vi "sim_pmt.vi"(4 "A":dbl=1.0, 6 "eff":dbl=0.25, 7 "N":i32=600, 8 "tau":dbl=142.0, 9 "sigma":dbl=10.0, 10 "dx":dbl=1.0 format="%#_13g", 11 "x0":dbl=-100.0) -> (2 "y":dbl[](array[numeric])=[1.9287498479639178e-22, 5.216736662027038e-22, 1.3969439431470991e-21, 3.703531977652345e-21, 9.72098502030078e-21, 2.5261637809256925e-20, 6.499347972070893e-20, 1.6555226620987744e-19, 4.175010055850514e-19, 1.04240617839016e-18, 2.576757109154981e-18, 6.306189893986447e-18, 1.5279799682873048e-17, 3.665433395601045e-17, 8.705426622296251e-17, 2.0469717131642043e-16, 4.765304735299088e-16, 1.0983141298285972e-15, 2.5062218871452745e-15, 5.6619955169489504e-15, 1.2664165549094176e-14, 2.804404738222797e-14, 6.148396412704756e-14, 1.3345660848219891e-13, 2.867975008888098e-13, 6.101936677605324e-13, 1.2853372251336503e-12, 2.680547637312607e-12, 5.5346100717010135e-12, 1.1313776200065328e-11, 2.289734845645553e-11, 4.5879624871392916e-11, 9.101470764487935e-11, 1.7875588711279812e-10, 3.475891281239922e-10, 6.691586091292782e-10, 1.2754076295260442e-09, 2.406722436301052e-09, 4.49634946228087e-09, 8.316702456828333e-09, 1.522997974471263e-08, 2.761242456828035e-08, 4.956405319172498e-08, 8.808179196460557e-08, 1.5497531357028967e-07, 2.699578503363014e-07, 4.6557157157830866e-07, 7.949393615349141e-07, 1.3438122776315214e-06, 2.2490559670323425e-06, 3.726653172078671e-06, 6.113567966371402e-06, 9.929504305851081e-06, 1.5966783897804747e-05, 2.5419346516199247e-05, 4.006529739295107e-05, 6.252150377482026e-05, 9.659341372218401e-05, 0.00014774836023203364, 0.00022374579372062055, 0.00033546262790251185, 0.0004979554215032735, 0.0007318024188804728, 0.0010647662366679205, 0.001533810679324463, 0.002187491118182885, 0.0030887154082367687, 0.004317840007633078, 0.005976022895005943, 0.008188701014374083, 0.011108996538242306, 0.014920786069067842, 0.019841094744370288, 0.026121409853918233, 0.034047454734599344, 0.04393693362340742, 0.056134762834133725, 0.07100535373963698, 0.08892161745938634, 0.11025052530448522, 0.1353352832366127, 0.1644744565771549, 0.19789869908361465, 0.23574607655586352, 0.27803730045319414, 0.32465246735834974, 0.37531109885139957, 0.42955735821073915, 0.4867522559599717, 0.5460744266397094, 0.6065306597126334, 0.6669768108584744, 0.7261490370736909, 0.7827045382418681, 0.835270211411272, 0.8824969025845955, 0.9231163463866358, 0.9559974818331, 0.9801986733067553, 0.9950124791926823, 1.25, 1.2432581004527816, 1.2267022272060057, 1.2007711933552672, 1.1661723547264784, 1.123847261749892, 1.0749268908206204, 1.0206794233182925, 0.9624539298340817, 0.9016234304988917, 0.8395306431895039, 0.7774393292469436, 0.7164935519020325, 0.657686441171688, 0.6018392825599493, 0.549590986148953, 0.5013973098231934, 0.4575386537187317, 0.4181348435183134, 0.3831650905736379, 0.35249125243750024, 0.32588259924293844, 0.3030404900932062, 0.2836216439816156, 0.267259015078684, 0.2535796182694965, 0.24221896870501314, 0.23283207711088139, 0.22510116680154815, 0.21874044249997526, 0.21349834548108462, 0.20915777967334567, 0.20553479803807054, 0.20247620846081113, 0.1998565045464241, 0.19757445935252493, 0.1955496479411705, 0.19371909445812904, 0.19203417601001516, 0.19045786174415458, 0.1889623224662098, 0.18752691382132963, 0.18613651360422623, 0.18478017971529853, 0.18345008797568668, 0.18214070677818295, 0.18084816685156144, 0.17956978795328984, 0.17830372904758776, 0.1770487337057488, 0.1758039475556503, 0.17456878927836056, 0.17334286072721433, 0.17212588516622737, 0.17091766540284734, 0.16971805578245663, 0.168526943698985, 0.16734423754450112, 0.16616985895450573, 0.1650037378796452, 0.16384580949201014, 0.162696012266431, 0.1615542868044931, 0.1604205751219807, 0.1592948202218085, 0.15817696584061583, 0.157066956299691, 0.1559647364178046, 0.15487025146033528, 0.15378344710941852, 0.1527042694461285, 0.15163266493947214, 0.1505685804391951, 0.14951196317070164, 0.1484627607311352, 0.14742092108609436, 0.14638639256669508, 0.14535912386682462, 0.14433906404050334, 0.14332616249931096, 0.14232036900985437, 0.14132163369126458, 0.14032990701271744, 0.1393451397909746, 0.1383672831879428, 0.1373962887082515, 0.13643210819684728, 0.13547469383660565, 0.1345239981459596, 0.13357997397654467, 0.13264257451086087, 0.13171175325995063, 0.13078746406109337, 0.1298696610755161, 0.12895829878612006, 0.12805333199522348, 0.12715471582231996, 0.12626240570185276, 0.12537635738100453, 0.12449652691750278, 0.12362287067744056, 0.12275534533311253, 0.12189390786086615, 0.12103851553896804, 0.12018912594548517, 0.1193456969561811, 0.11850818674242683, 0.1176765537691264, 0.11685075679265702, 0.1160307548588236, 0.11521650730082776, 0.11440797373725096, 0.11360511407005193, 0.1128078884825779, 0.11201625743759017, 0.11123018167530312, 0.11044962221143731, 0.10967454033528602, 0.10890489760779555, 0.1081406558596588, 0.10738177718942235, 0.1066282239616068, 0.10587995880484032, 0.10513694461000518, 0.10439914452839749, 0.10366652196989969, 0.10293904060116589, 0.10221666434382001, 0.10149935737266652, 0.10078708411391372, 0.10007980924340955, 0.0993774976848897, 0.09868011460823806, 0.09798762542775939, 0.0972999958004641, 0.09661719162436501, 0.09593917903678618, 0.09526592441268349, 0.09459739436297705, 0.09393355573289539, 0.09327437560033107, 0.0926198212742081, 0.09196986029286058, 0.09132446042242282, 0.09068358965523078, 0.09004721620823468, 0.08941530852142278, 0.08878783525625616, 0.0881647652941146, 0.08754606773475325, 0.0869317118947702, 0.08632166730608473, 0.08571590371442639, 0.0851143910778345, 0.08451709956516827, 0.08392399955462743, 0.0833350616322831, 0.0827502565906191, 0.08216955542708343, 0.08159292934264993, 0.08102034974039005, 0.08045178822405458, 0.07988721659666545, 0.0793266068591173, 0.07876993120878888, 0.0782171620381643, 0.07766827193346378, 0.07712323367328416, 0.07658202022724891, 0.07604460475466757, 0.07551096060320459, 0.07498106130755759, 0.07445488058814488, 0.0739323923498021, 0.07341357068048812, 0.07289838984999991, 0.07238682430869656, 0.07187884868623211, 0.07137443779029741, 0.07087356660537074, 0.07037621029147711, 0.0698823441829565, 0.06939194378724046, 0.06890498478363756, 0.06842144302212716, 0.06794129452216174, 0.06746451547147767, 0.06699108222491419, 0.06652097130324086, 0.06605415939199304, 0.0655906233403157, 0.06513034015981535, 0.0646732870234198, 0.06421944126424624, 0.06376878037447704, 0.0633212820042435, 0.06287692396051747, 0.06243568420601071, 0.06199754085808197, 0.06156247218765177, 0.06113045661812477, 0.06070147272431971, 0.06027549923140684, 0.05985251501385289, 0.05943249909437331, 0.05901543064289194, 0.05860128897550802, 0.05819005355347037, 0.05778170398215878, 0.05737622001007262, 0.05697358152782646, 0.056573768567152766, 0.05617676129991164, 0.055782540037107455, 0.0553910852279124, 0.05500237745869686, 0.05461639745206672, 0.05423312606590721, 0.05385254429243366, 0.05347463325724882, 0.053099374218406784, 0.052726748565483546, 0.052356737818654034, 0.051989323627775606, 0.05162448777147804, 0.05126221215625983, 0.05090247881559093, 0.05054526990902163, 0.050190567721297895, 0.04983835466148272, 0.04948861326208375, 0.04914132617818706, 0.048796476186596896, 0.04845404618498154, 0.04811401919102513, 0.04777637834158547, 0.04744110689185774, 0.04710818821454399, 0.04677760579902863, 0.04644934325055953, 0.04612338428943498, 0.04579971275019635, 0.04547831258082632, 0.04515916784195286, 0.044842262706058726, 0.044527581456696504, 0.04421510848770919, 0.04390482830245621, 0.043596725513044915, 0.0432907848395674, 0.04298699110934278, 0.04268532925616464, 0.042385784319553914, 0.04208834144401693, 0.04179298587830866, 0.041499702974701146, 0.04120847818825709, 0.040919297076108516, 0.04063214529674048, 0.04034700860927983, 0.04006387287278897, 0.03978272404556454, 0.039503548184441024, 0.03922633144409931, 0.03895106007637999, 0.03867772042960159, 0.03840629894788351, 0.03813678217047375, 0.03786915673108132, 0.0376034093572134, 0.037339526869517074, 0.037077496181125734, 0.03681730429701006, 0.03655893831333352, 0.036302385416812494, 0.03604763288408073, 0.03579466808105841, 0.035543478462325556, 0.035294051570499856, 0.03504637503561887, 0.03480043657452655, 0.03455622399026408, 0.03431372517146501, 0.034072928091754544, 0.033833820809153176, 0.0335963914654844, 0.03336062828578669, 0.03312651957772941, 0.032894053731033115, 0.032663219216893594, 0.032434004587410255, 0.03220639847501826, 0.03198038959192488, 0.031755966729549605, 0.03153311875796834, 0.03131183462536134, 0.031092103357465258, 0.030873914057028714, 0.030657255903272018, 0.03044211815135042, 0.030228490131821318, 0.030016361250115038, 0.029805720986009508, 0.029596558893108423, 0.029388864598323267, 0.029182627801358774, 0.028977838274202215, 0.028774485860616032, 0.028572560475634265, 0.02837205210506234, 0.028172950804980418, 0.02797524670125031, 0.027778929989025692, 0.02758399093226594, 0.0273904198632532, 0.027198207182113018, 0.027007343356338146, 0.02681781892031591, 0.02662962447485866, 0.02644275068673773, 0.026257188288220486, 0.02607292807661079, 0.025889960913792507, 0.025708277725776434, 0.02552786950225016, 0.02534872729613133, 0.02517084222312382, 0.024994205461277244, 0.02481880825054933, 0.024644641892371585, 0.024471697749217796, 0.02429996724417578, 0.024129441860521905, 0.02396011314129881, 0.02379197268889597, 0.023625012164633166, 0.023459223288347052, 0.0232945978379804, 0.023131127649174438, 0.02296880461486386, 0.02280762068487486, 0.02264756786552579, 0.02248863821923084, 0.02233082386410628, 0.022174116973579655, 0.022018509776001564, 0.02186399455426031, 0.0217105636453991, 0.0215582094402361, 0.021406924382986983, 0.02125670097089028, 0.021107531753835243, 0.020959409333992412, 0.02081232636544667, 0.02066627555383301, 0.0205212496559747, 0.02037724147952414, 0.02023424388260614, 0.02009224977346369, 0.019951252110106326, 0.019811243899960838, 0.01967221819952452, 0.019534168114020773, 0.019397086797057234, 0.01926096745028616, 0.01912580332306735, 0.018991587712133294, 0.018858313961256788, 0.018725975460920773, 0.018594565647990603, 0.0184640780053885, 0.018334506061770412, 0.018205843391205, 0.01807808361285503, 0.017951220390660858, 0.017825247433026267, 0.017700158492506373, 0.017575947365497866, 0.017452607891931284, 0.017330133954965566, 0.01720851948068467, 0.01708775843779634, 0.016967844837333025, 0.01684877273235481, 0.016730536217654562, 0.01661312942946498, 0.016496546545167894, 0.016380781783005383, 0.016265829401793153, 0.016151683700635713, 0.016038339018643728, 0.015925789734653202, 0.015814030266946784, 0.015703055072976865, 0.01559285864909078, 0.015483435530257805, 0.015374780289798173, 0.0152668875391139, 0.015159751927421592, 0.015053368141487035, 0.014947730905361738, 0.014842834980121237, 0.014738675163605318, 0.014635246290159984, 0.014532543230381306, 0.01443056089086103, 0.014329294213933945, 0.01422873817742711, 0.014128887794410737, 0.014029738112950907, 0.013931284215863957, 0.013833521220472652, 0.013736444278363994, 0.013640048575148823, 0.013544329330222999, 0.01344928179653037, 0.013354901260327297, 0.01326118304094893, 0.013168122490577033, 0.013075714994009524, 0.012983955968431552, 0.012892840863188258, 0.012802365159559048, 0.012712524370533544, 0.012623314040589001, 0.012534729745469403, 0.012446767091965986, 0.012359421717699416, 0.012272689290903417, 0.01218656551020994, 0.01210104610443586, 0.01201612683237113, 0.011931803482568481, 0.011848071873134509, 0.011764927851522337, 0.011682367294325624, 0.011600386107074118, 0.01151898022403055, 0.011438145607989045, 0.01135787825007486, 0.011278174169545612, 0.011199029413593813, 0.011120440057150885, 0.011042402202692456, 0.010964911980045108, 0.010887965546194409, 0.010811559085094348, 0.010735688807478062, 0.010660350950669943, 0.010585541778398995, 0.010511257580613572, 0.010437494673297378, 0.010364249398286732, 0.0102915181230892, 0.010219297240703392, 0.010147583169440127, 0.010076372352744762, 0.010005661259020845, 0.009935446381454943, 0.00986572423784275, 0.009796491370416367, 0.00972774434567285, 0.009659479754203892, 0.009591694210526785, 0.009524384352916472, 0.009457546843238874, 0.009391178366785295, 0.009325275632108079, 0.009259835370857335, 0.009194854337618885, 0.00913032930975327, 0.009066257087235975, 0.009002634492498687, 0.00893945837027174, 0.008876725587427605, 0.00881443303282554, 0.008752577617157267, 0.008691156272793776, 0.008630165953633199, 0.008569603634949718, 0.008509466313243591, 0.008449751006092163, 0.00839045475200199, 0.008331574610261941, 0.00827310766079738, 0.008215051004025326, 0.008157401760710677, 0.008100157071823395, 0.008043314098396741, 0.007986870021386453, 0.007930822041530968, 0.007875167379212573, 0.007819903274319572, 0.007765026986109383, 0.00771053579307264, 0.007656426992798195, 0.007602697901839126, 0.007549345855579625, 0.007496368208102875, 0.007443762332059822], 3 "x":dbl[](array[numeric])=[-100.0, -99.0, -98.0, -97.0, -96.0, -95.0, -94.0, -93.0, -92.0, -91.0, -90.0, -89.0, -88.0, -87.0, -86.0, -85.0, -84.0, -83.0, -82.0, -81.0, -80.0, -79.0, -78.0, -77.0, -76.0, -75.0, -74.0, -73.0, -72.0, -71.0, -70.0, -69.0, -68.0, -67.0, -66.0, -65.0, -64.0, -63.0, -62.0, -61.0, -60.0, -59.0, -58.0, -57.0, -56.0, -55.0, -54.0, -53.0, -52.0, -51.0, -50.0, -49.0, -48.0, -47.0, -46.0, -45.0, -44.0, -43.0, -42.0, -41.0, -40.0, -39.0, -38.0, -37.0, -36.0, -35.0, -34.0, -33.0, -32.0, -31.0, -30.0, -29.0, -28.0, -27.0, -26.0, -25.0, -24.0, -23.0, -22.0, -21.0, -20.0, -19.0, -18.0, -17.0, -16.0, -15.0, -14.0, -13.0, -12.0, -11.0, -10.0, -9.0, -8.0, -7.0, -6.0, -5.0, -4.0, -3.0, -2.0, -1.0, 0.0, 1.0, 2.0, 3.0, 4.0, 5.0, 6.0, 7.0, 8.0, 9.0, 10.0, 11.0, 12.0, 13.0, 14.0, 15.0, 16.0, 17.0, 18.0, 19.0, 20.0, 21.0, 22.0, 23.0, 24.0, 25.0, 26.0, 27.0, 28.0, 29.0, 30.0, 31.0, 32.0, 33.0, 34.0, 35.0, 36.0, 37.0, 38.0, 39.0, 40.0, 41.0, 42.0, 43.0, 44.0, 45.0, 46.0, 47.0, 48.0, 49.0, 50.0, 51.0, 52.0, 53.0, 54.0, 55.0, 56.0, 57.0, 58.0, 59.0, 60.0, 61.0, 62.0, 63.0, 64.0, 65.0, 66.0, 67.0, 68.0, 69.0, 70.0, 71.0, 72.0, 73.0, 74.0, 75.0, 76.0, 77.0, 78.0, 79.0, 80.0, 81.0, 82.0, 83.0, 84.0, 85.0, 86.0, 87.0, 88.0, 89.0, 90.0, 91.0, 92.0, 93.0, 94.0, 95.0, 96.0, 97.0, 98.0, 99.0, 100.0, 101.0, 102.0, 103.0, 104.0, 105.0, 106.0, 107.0, 108.0, 109.0, 110.0, 111.0, 112.0, 113.0, 114.0, 115.0, 116.0, 117.0, 118.0, 119.0, 120.0, 121.0, 122.0, 123.0, 124.0, 125.0, 126.0, 127.0, 128.0, 129.0, 130.0, 131.0, 132.0, 133.0, 134.0, 135.0, 136.0, 137.0, 138.0, 139.0, 140.0, 141.0, 142.0, 143.0, 144.0, 145.0, 146.0, 147.0, 148.0, 149.0, 150.0, 151.0, 152.0, 153.0, 154.0, 155.0, 156.0, 157.0, 158.0, 159.0, 160.0, 161.0, 162.0, 163.0, 164.0, 165.0, 166.0, 167.0, 168.0, 169.0, 170.0, 171.0, 172.0, 173.0, 174.0, 175.0, 176.0, 177.0, 178.0, 179.0, 180.0, 181.0, 182.0, 183.0, 184.0, 185.0, 186.0, 187.0, 188.0, 189.0, 190.0, 191.0, 192.0, 193.0, 194.0, 195.0, 196.0, 197.0, 198.0, 199.0, 200.0, 201.0, 202.0, 203.0, 204.0, 205.0, 206.0, 207.0, 208.0, 209.0, 210.0, 211.0, 212.0, 213.0, 214.0, 215.0, 216.0, 217.0, 218.0, 219.0, 220.0, 221.0, 222.0, 223.0, 224.0, 225.0, 226.0, 227.0, 228.0, 229.0, 230.0, 231.0, 232.0, 233.0, 234.0, 235.0, 236.0, 237.0, 238.0, 239.0, 240.0, 241.0, 242.0, 243.0, 244.0, 245.0, 246.0, 247.0, 248.0, 249.0, 250.0, 251.0, 252.0, 253.0, 254.0, 255.0, 256.0, 257.0, 258.0, 259.0, 260.0, 261.0, 262.0, 263.0, 264.0, 265.0, 266.0, 267.0, 268.0, 269.0, 270.0, 271.0, 272.0, 273.0, 274.0, 275.0, 276.0, 277.0, 278.0, 279.0, 280.0, 281.0, 282.0, 283.0, 284.0, 285.0, 286.0, 287.0, 288.0, 289.0, 290.0, 291.0, 292.0, 293.0, 294.0, 295.0, 296.0, 297.0, 298.0, 299.0, 300.0, 301.0, 302.0, 303.0, 304.0, 305.0, 306.0, 307.0, 308.0, 309.0, 310.0, 311.0, 312.0, 313.0, 314.0, 315.0, 316.0, 317.0, 318.0, 319.0, 320.0, 321.0, 322.0, 323.0, 324.0, 325.0, 326.0, 327.0, 328.0, 329.0, 330.0, 331.0, 332.0, 333.0, 334.0, 335.0, 336.0, 337.0, 338.0, 339.0, 340.0, 341.0, 342.0, 343.0, 344.0, 345.0, 346.0, 347.0, 348.0, 349.0, 350.0, 351.0, 352.0, 353.0, 354.0, 355.0, 356.0, 357.0, 358.0, 359.0, 360.0, 361.0, 362.0, 363.0, 364.0, 365.0, 366.0, 367.0, 368.0, 369.0, 370.0, 371.0, 372.0, 373.0, 374.0, 375.0, 376.0, 377.0, 378.0, 379.0, 380.0, 381.0, 382.0, 383.0, 384.0, 385.0, 386.0, 387.0, 388.0, 389.0, 390.0, 391.0, 392.0, 393.0, 394.0, 395.0, 396.0, 397.0, 398.0, 399.0, 400.0, 401.0, 402.0, 403.0, 404.0, 405.0, 406.0, 407.0, 408.0, 409.0, 410.0, 411.0, 412.0, 413.0, 414.0, 415.0, 416.0, 417.0, 418.0, 419.0, 420.0, 421.0, 422.0, 423.0, 424.0, 425.0, 426.0, 427.0, 428.0, 429.0, 430.0, 431.0, 432.0, 433.0, 434.0, 435.0, 436.0, 437.0, 438.0, 439.0, 440.0, 441.0, 442.0, 443.0, 444.0, 445.0, 446.0, 447.0, 448.0, 449.0, 450.0, 451.0, 452.0, 453.0, 454.0, 455.0, 456.0, 457.0, 458.0, 459.0, 460.0, 461.0, 462.0, 463.0, 464.0, 465.0, 466.0, 467.0, 468.0, 469.0, 470.0, 471.0, 472.0, 473.0, 474.0, 475.0, 476.0, 477.0, 478.0, 479.0, 480.0, 481.0, 482.0, 483.0, 484.0, 485.0, 486.0, 487.0, 488.0, 489.0, 490.0, 491.0, 492.0, 493.0, 494.0, 495.0, 496.0, 497.0, 498.0, 499.0])   [LabVIEW 2015, in "daq_simulate.lvlib"]
uses:
  daq_simulate.lvlib
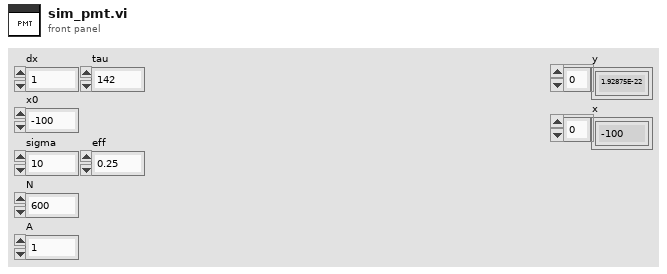
[diagram p1: front panel]
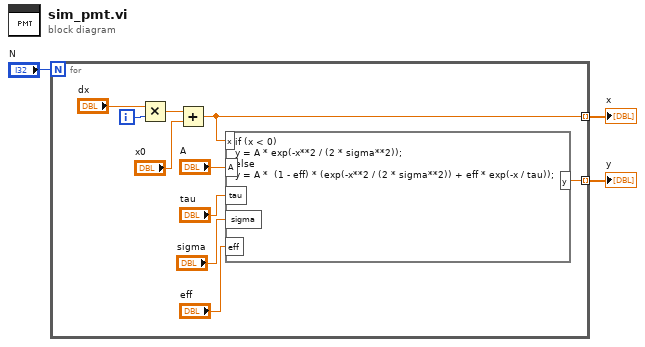
[diagram p0: block diagram]
diagram:
  n1 = for {
    N: "N" -> [_]
    tunnel: [w9] -> w1 mode=indexing
    tunnel: [w6] -> w2 mode=indexing
    i -> [w13]
    n2 = Multiply(x="dx", y=w13) -> (x*y=w10:dbl)
    n3 = Add(x=w10, y="x0") -> (x+y=w6:dbl)
    n4 = formula code="if (x < 0)\ny = A * exp(-x**2 / (2 * sigma**2));\nelse\ny = A *  (1 - eff) * (exp(-x**2 / (2 * sigma**2)) + eff * exp(-x / tau));"("x"=w6, "tau"="tau", "sigma"="sigma", "eff"="eff", "A"="A") -> ("y"=w9:dbl)
  }
  "y" <- w1
  "x" <- w2
